vi "Kinect Handle FGV.vi"(7 "Handle Command":T1, 10 "Context Handle In":i64, 11 "Kinect Handle In":i64) -> (2 "Context Handle Out":i64, 3 "Kinect Handle Out":i64)   [LabVIEW 2015]
uses:
  TypeDefs Host/Handle Enum.ctl
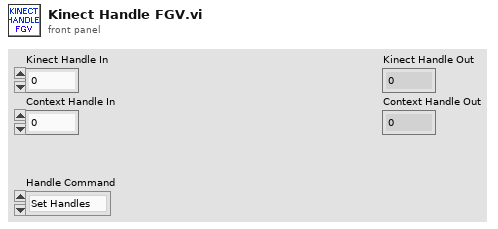
[diagram p1: front panel]
types:
  T1 = typedef "Handle Enum.ctl" = enum16{"Set Handles", "Get Handles"}
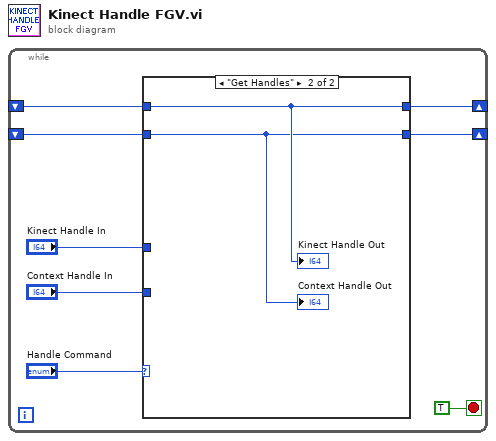
[diagram p0: block diagram]
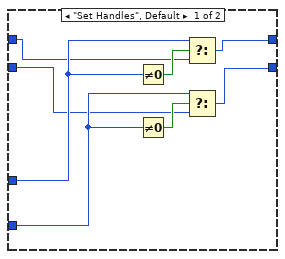
[diagram p2: hidden frame]
diagram:
  n1 = while {
    shift-right: [w4] -> _
    shift-left: _ -> [w3]
    shift-right: [w1] -> _
    shift-left: _ -> [w2]
    stop <- TRUE stop-if-true
    n2 = case shown="\"Get Handles\"" "Handle Command" {
      tunnel: "Kinect Handle In" -> [w15 _]
      tunnel: "Context Handle In" -> [w11 _]
      tunnel: [w13 w18] -> w4
      tunnel: w3 -> [w14 w18]
      tunnel: w2 -> [w10 w17]
      tunnel: [w9 w17] -> w1
      frame "Set Handles", Default {
        n3 = Not Equal To 0?(x=w15) -> (x != 0?=w16:bool)
        n4 = Not Equal To 0?(x=w11) -> (x != 0?=w12:bool)
        n5 = Select(t=w15, s=w16, f=w14) -> (s? t:f=w13:i64)
        n6 = Select(t=w11, s=w12, f=w10) -> (s? t:f=w9:i64)
      }
      frame "Get Handles" {
        "Kinect Handle Out" <- w18
        "Context Handle Out" <- w17
      }
    }
  }
